vi "main.vi"() -> ()   [LabVIEW 2016]
doc: "Ezt a VI-t kell elindítani."
uses:
  adat.ctl
  <vilib>/Utility/file.llb/Write Delimited Spreadsheet (string).vi
panel:
  in  "1":enum32{""}(tab)
  in  "2":T1(tab)
  out "Waveform Graph":dbl[][](graph)
  out "XY Graph":cluster{dbl[], dbl[]}[](graph)
  out "Waveform Graph 2":dbl[][](graph)
  out "XY Graph 3":cluster{dbl[], dbl[]}[](graph)
  out "XY Graph 4":cluster{dbl[], dbl[]}[](graph)
  out "XY Graph 5":cluster{dbl[], dbl[]}[](graph)
  in  "Kiértékelés indítása":bool
  in  "Program leállítása":bool
  in  "Kilépés a programból":bool
  in  "Eredmények mentése":bool
  in  "Inicializálás":bool
  in  "Fájlbeolvasás":bool
  in  "Paraméterek betöltése":bool
  in  "Paraméterek mentése":bool
  in  "Kezelõpult":T2={"Filt_alsó"=750.0, "Filt_felsõ"=7400.0, "Optikai elem hossza (km)"=0.000445, "Referencia hullámhossz (nm)"=800.0, " Illesztendõ polinom fokszáma"=7, "Megjegyzések"="**********"}
  # "Az Ocean Optics spektográffal kapott 1D-s \nspektrális interferogramok FT alapú kiértékelése\n\nLabview-ban implementálta:\nTari Balázs"
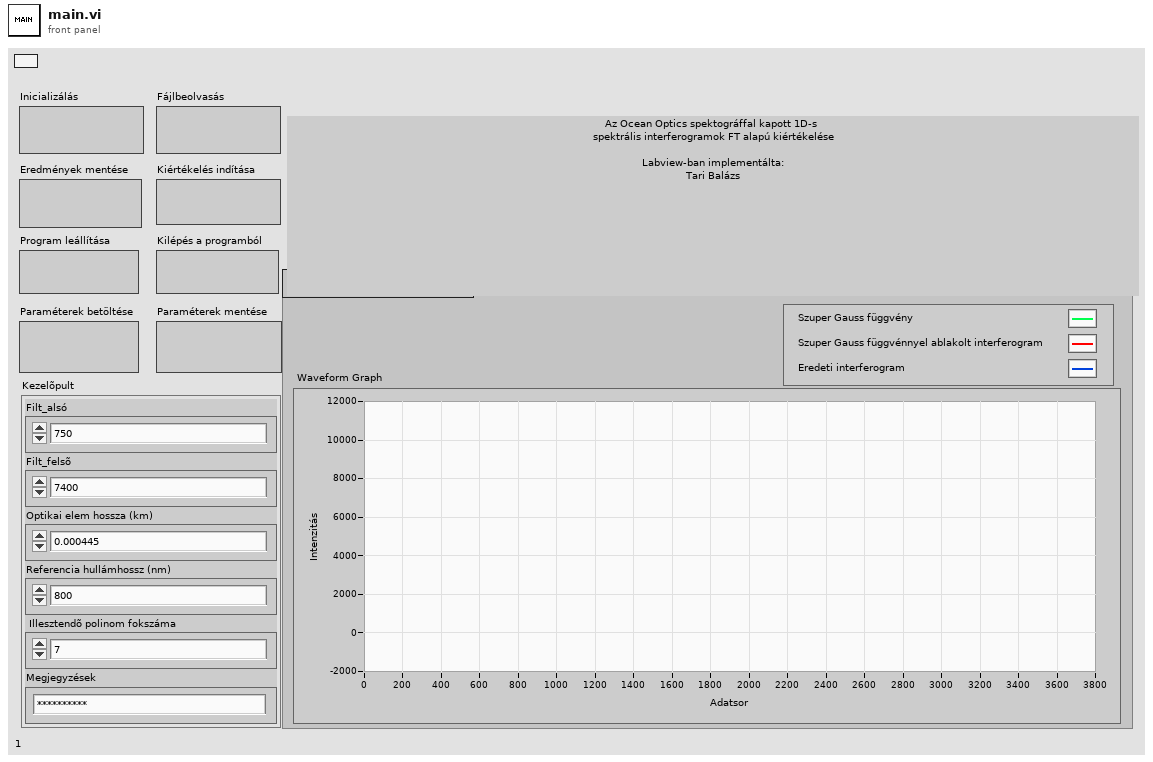
[diagram p1: front panel]
types:
  T1 = enum32{"Eredeti és módosított interferogram", "Megfordított interpolált és ablakolt interferogram", "Spektrum", "Fázis", "Fázisok összehasonlítása", "Diszperzió"}
  T2 = typedef "kezelõpult.ctl" = cluster{"Filt_alsó":dbl, "Filt_felsõ":dbl, "Optikai elem hossza (km)":dbl, "Referencia hullámhossz (nm)":dbl, " Illesztendõ polinom fokszáma":i32, "Megjegyzések":string}
  T3 = typedef "adat.ctl" = cluster{"Inicializálás":path, "Fájlbeolvasás":path, "Ix":dbl[], "dw":dbl, "Nw1":dbl, "Nw2":dbl, "FFT {X}":cdb[], "eredmények mentése":path}
  T4 = typedef "állapotok.ctl" = enum16{"init", "idle", "data load, filter, analysis", "filter", "analysis", "save", "save parameters", "load parameters", "stop"}
  T5 = enum16{"open", "replace", "create", "open or create", "replace or create", "replace or create with confirmation"}
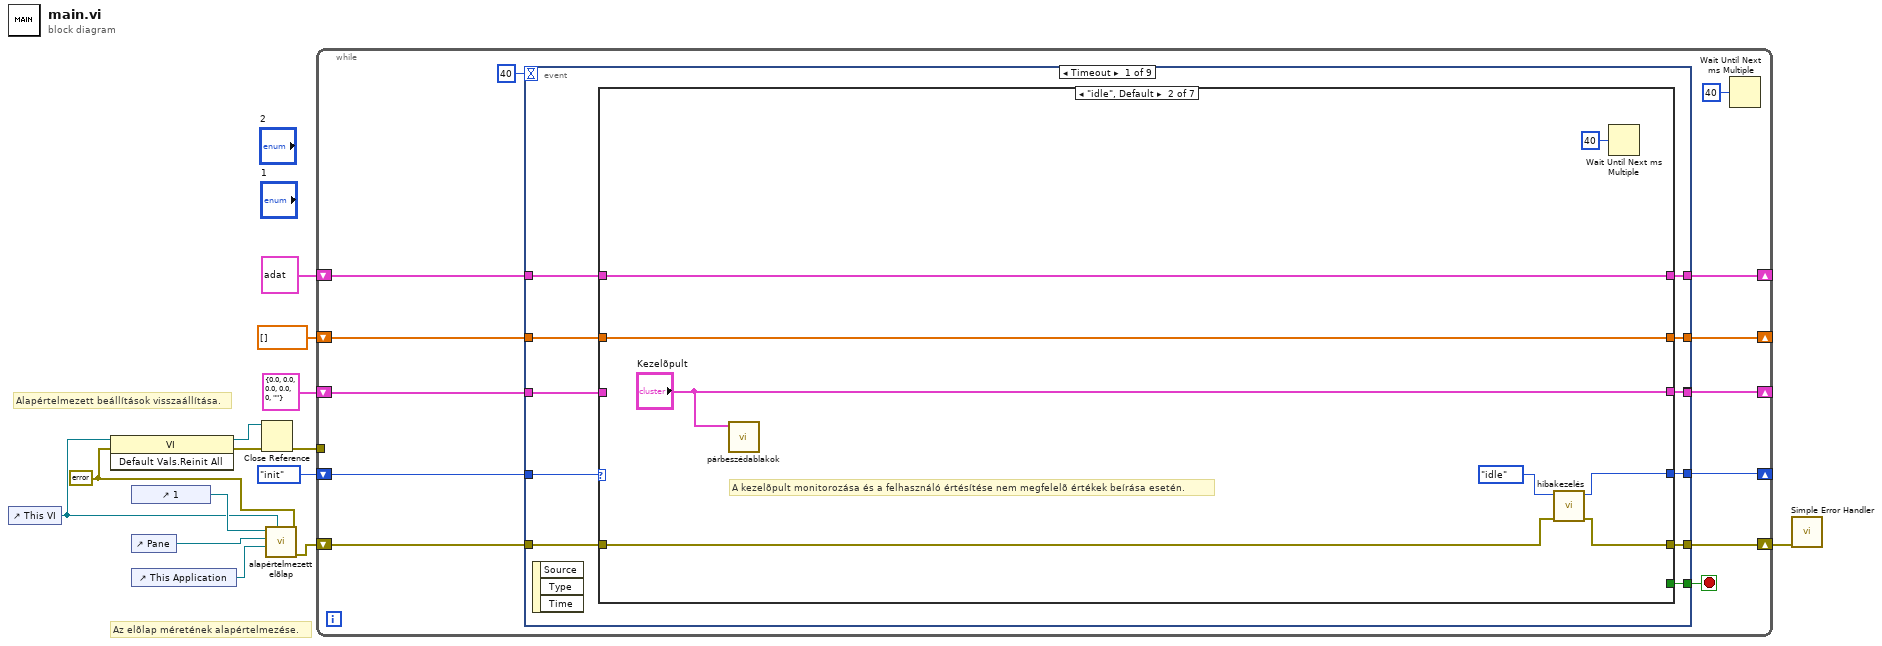
[diagram p0: block diagram]
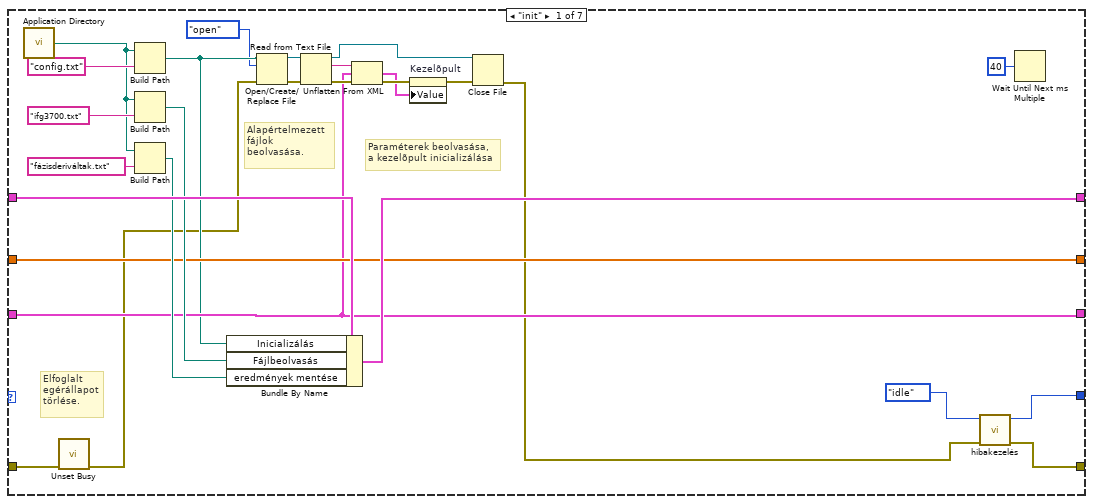
[diagram p2: hidden frame]
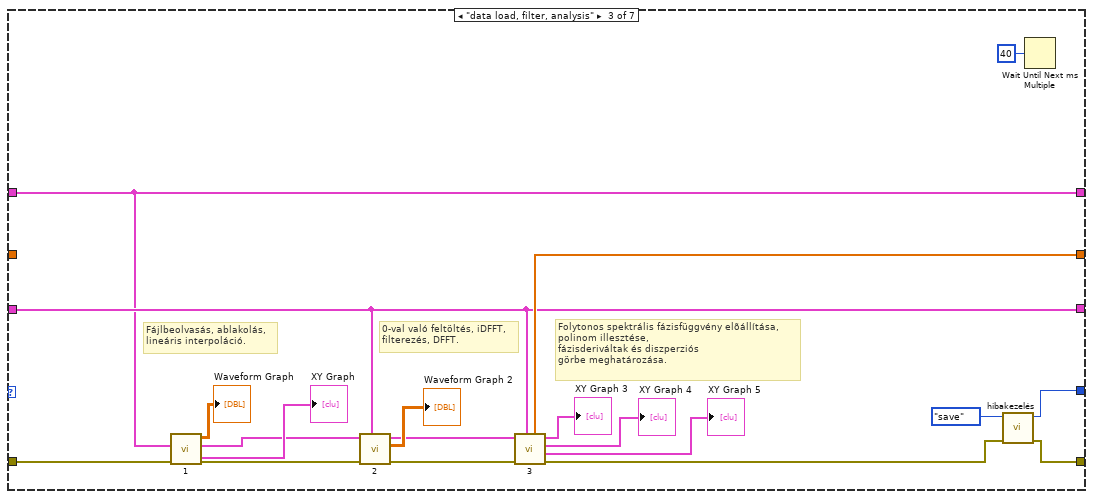
[diagram p3: hidden frame]
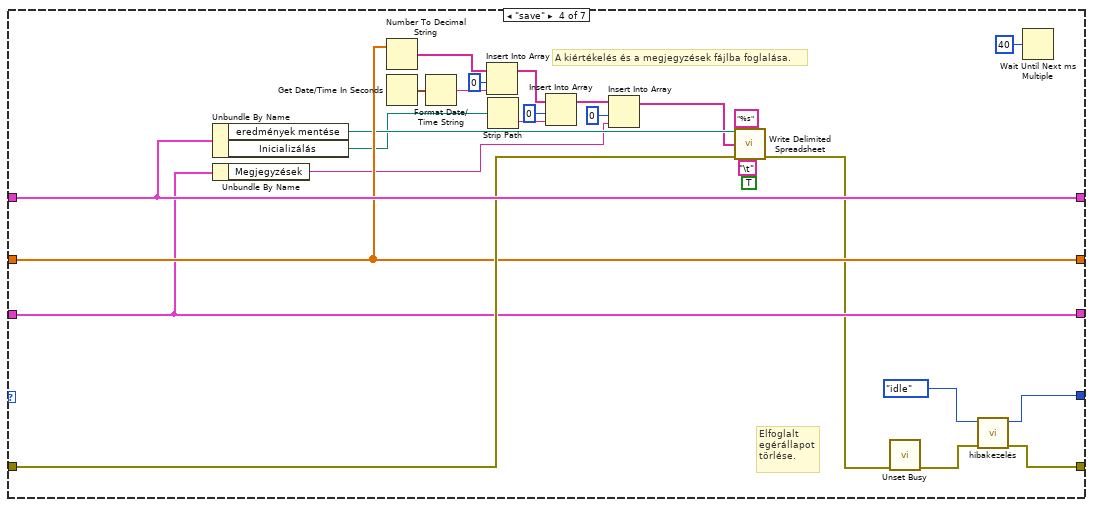
[diagram p4: hidden frame]
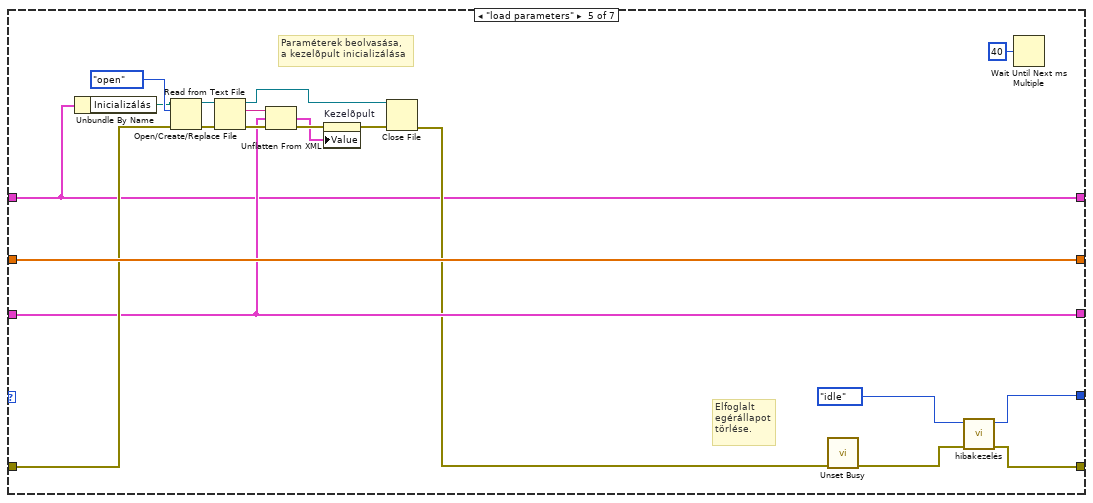
[diagram p5: hidden frame]
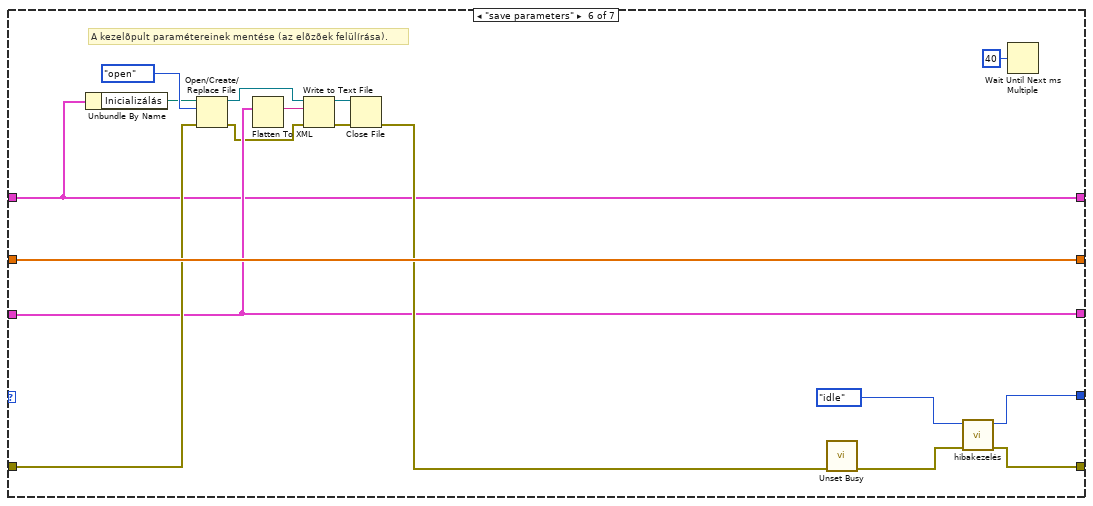
[diagram p6: hidden frame]
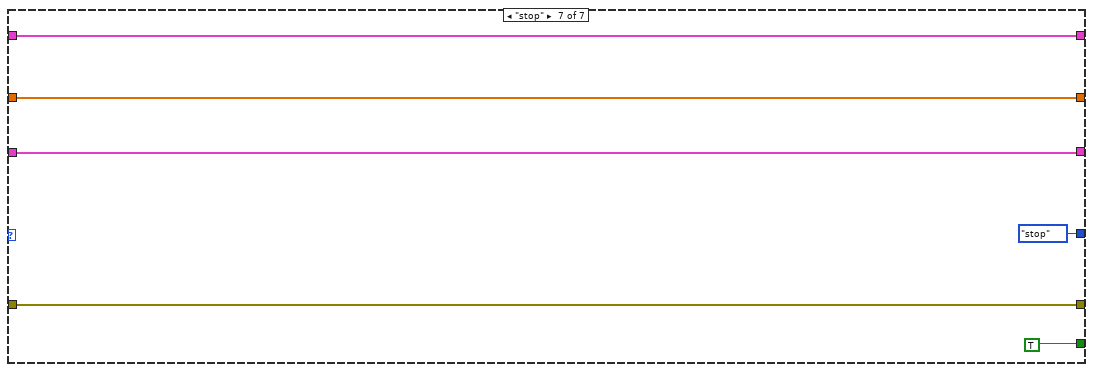
[diagram p7: hidden frame]
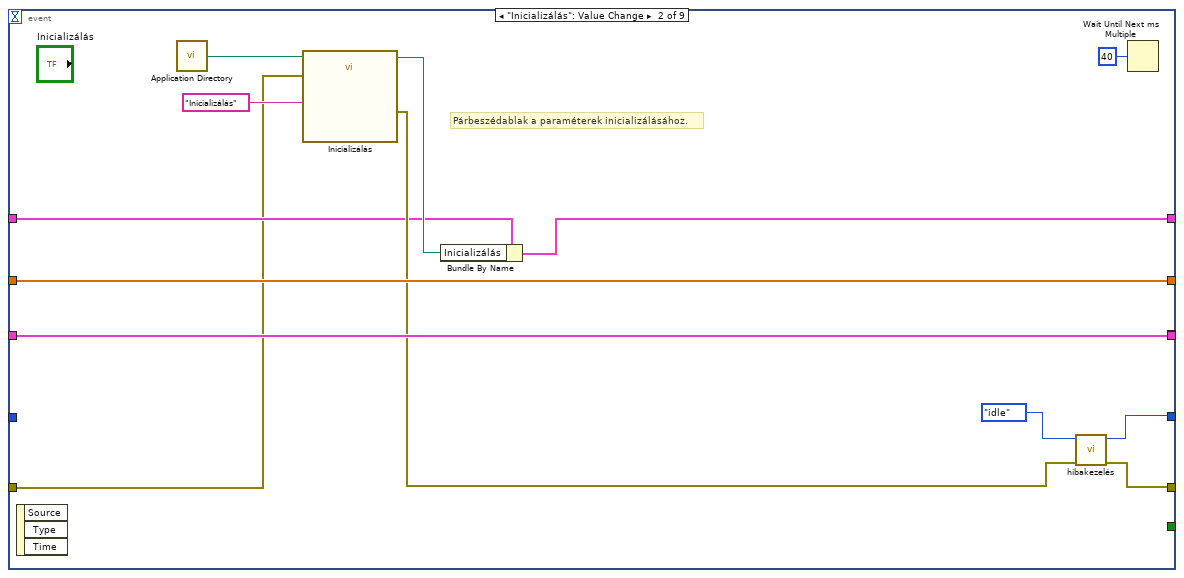
[diagram p8: hidden frame]
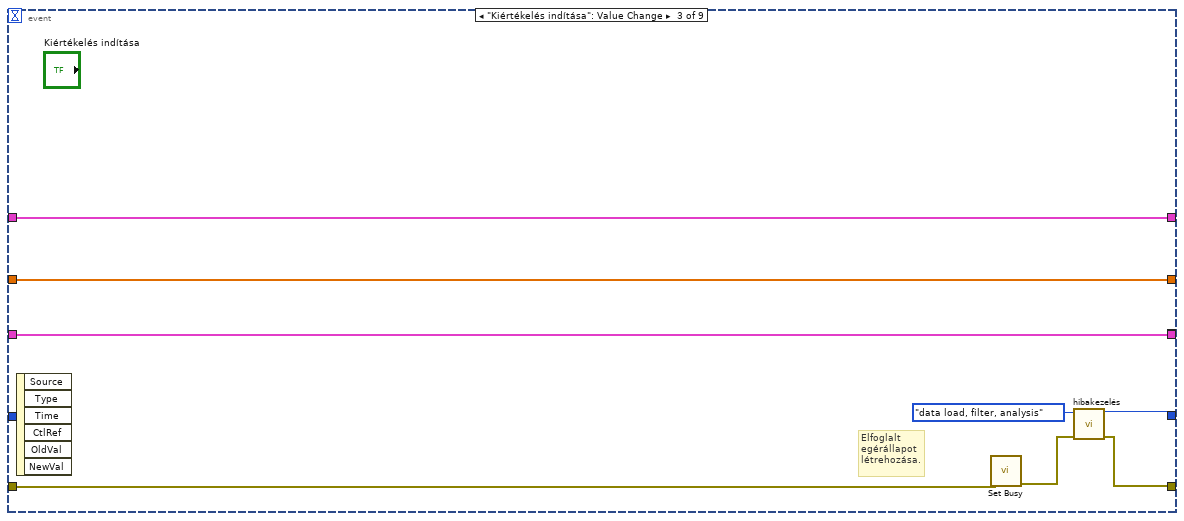
[diagram p9: hidden frame]
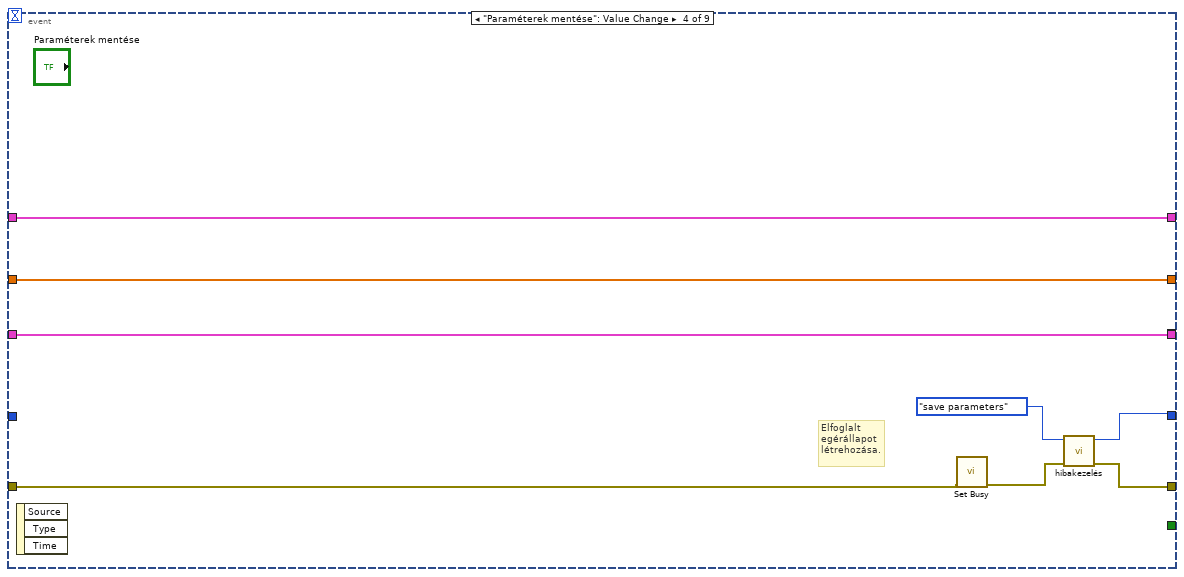
[diagram p10: hidden frame]
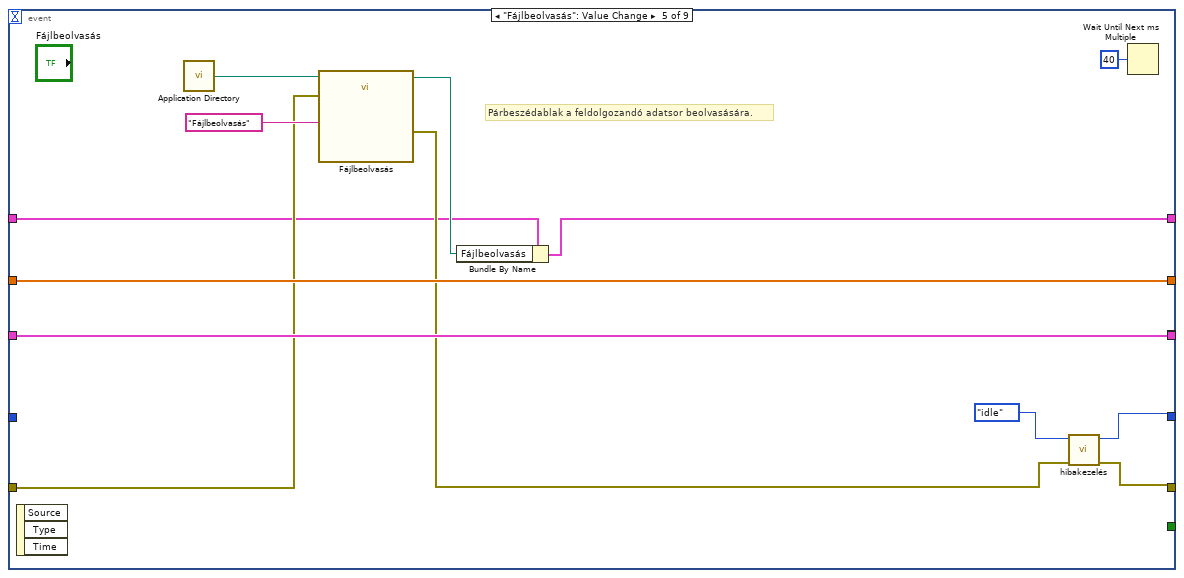
[diagram p11: hidden frame]
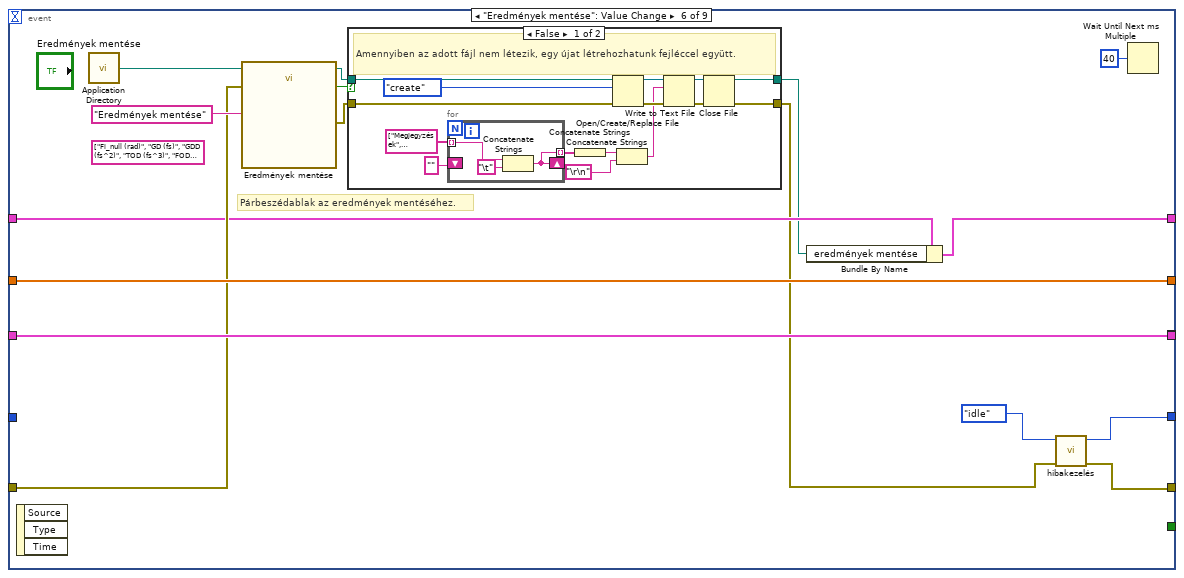
[diagram p12: hidden frame]
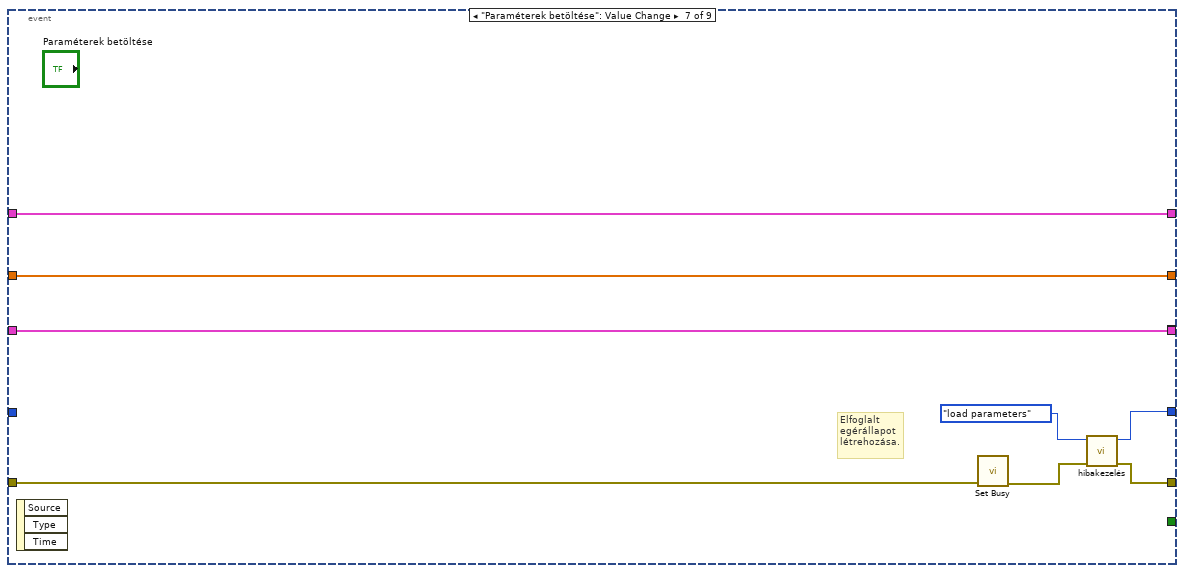
[diagram p14: hidden frame]
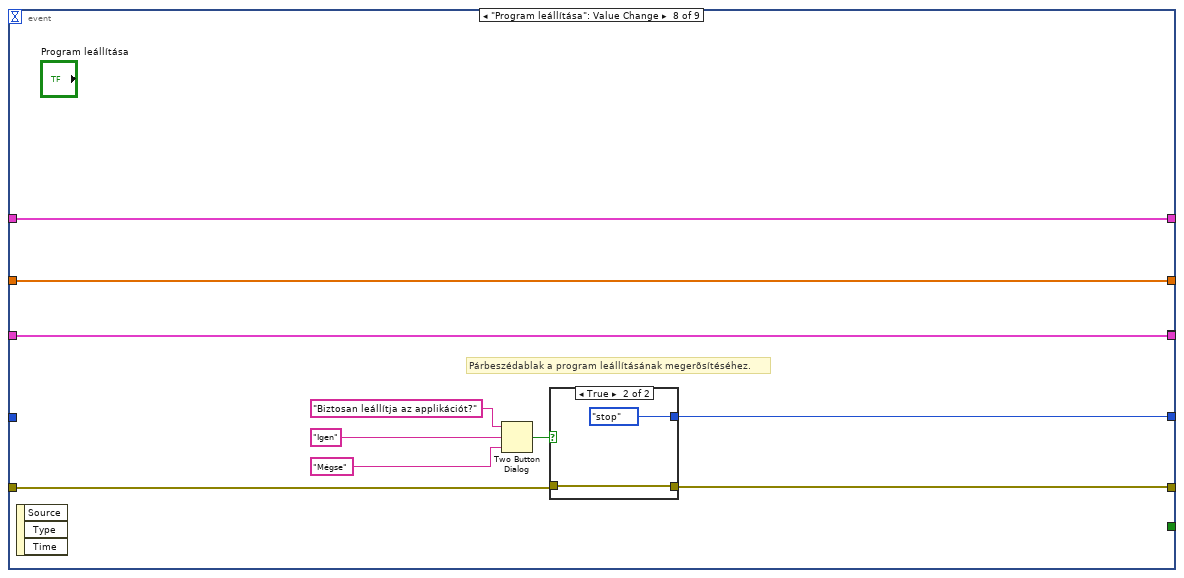
[diagram p15: hidden frame]
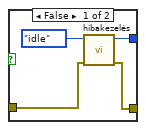
[diagram p16: hidden frame]
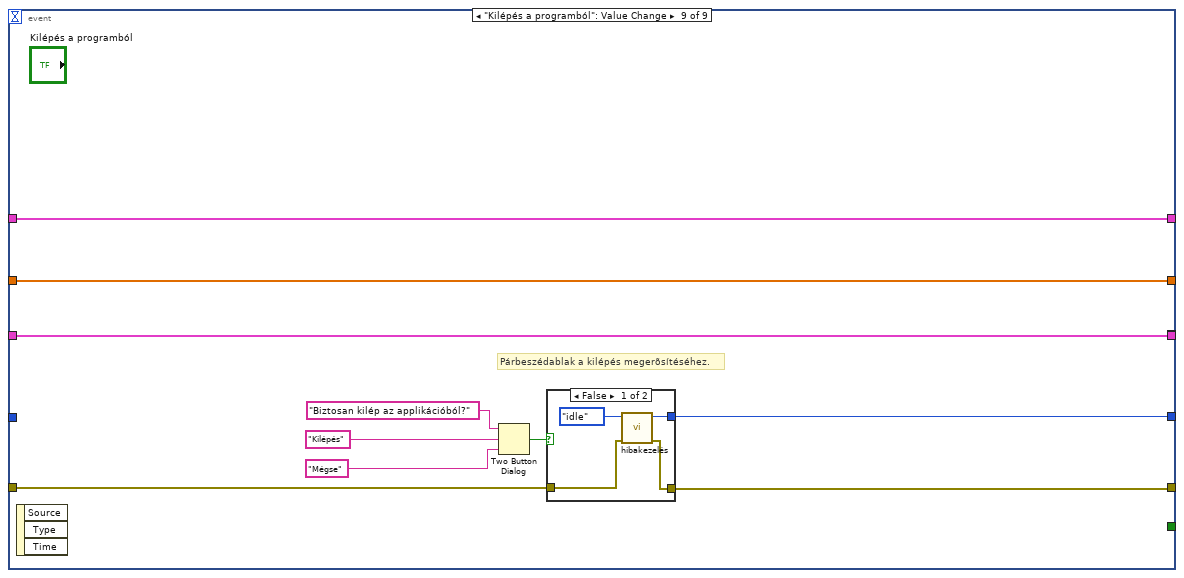
[diagram p17: hidden frame]
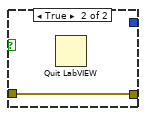
[diagram p18: hidden frame]
diagram:
  w6 = errorcluster {"status"=FALSE, "code"=0, "source"=""} ("error constant")
  # "Az elõlap méretének alapértelmezése."
  # "Alapértelmezett beállítások visszaállítása."
  n1 = control-ref of="This VI"() -> (w5:refnum<vi>)
  n2 = invoke class="VI" method="Default Vals.Reinit All"(reference=w5, error in=w6) -> (reference out=w3:refnum<vi>, error out=w4:errorcluster)  [unwired: 1 in, 1 out]
  n3 = control-ref of="1"() -> (w8:refnum<vi>)
  n4 = control-ref of="Pane"() -> (w7:refnum<vi>)
  n5 = control-ref of="This Application"() -> (w12:refnum<vi>)
  n6 = Close Reference(reference=w3, error in (no error)=w4) -> (error out=w1:errorcluster)
  n7 = call "alapértelmezett elõlap.vi"("error in (no error)"=w6, "VI Reference"=w5, "Application reference"=w12, "Pane Control"=w7, "TabControl in"=w8) -> ("error out"=w2:errorcluster)  [unwired: 6 in]
  n8 = while {
    shift-right: [w27] -> _
    shift-left: állapotok."init" -> [w17]
    shift-right: [w24] -> w11
    shift-left: w2 -> [w16]
    shift-right: [w23] -> _
    shift-left: T2 {"Filt_alsó"=0.0, "Filt_felsõ"=0.0, "Optikai elem hossza (km)"=0.0, "Referencia hullámhossz (nm)"=0.0, " Illesztendõ polinom fokszáma"=0, "Megjegyzések"=""} ("Kezelõpult") -> [w21]
    shift-right: [w20] -> _
    shift-left: T3 {"Inicializálás"=path "", "Fájlbeolvasás"=path "", "Ix"=[], "dw"=0.0, "Nw1"=0.0, "Nw2"=0.0, "FFT {X}"=[], "eredmények mentése"=path ""} ("adat") -> [w22]
    shift-right: [w19] -> _
    shift-left: dbl[] [] ("Fázisderiváltak") -> [w18]
    tunnel: w1 -> [_]
    stop <- w26 stop-if-true
    n9 = event shown="[0] Timeout" {
      selector: _ -> [_ _ _ _ _ _ _ _ _]
      dyn-events: _ -> [_ _ _ _ _ _ _ _ _]
      timeout: 40 -> [_ _ _ _ _ _ _ _ _]
      tunnel: w17 -> [w38 _ _ _ _ _ _ _ _]
      tunnel: [w37 w172 w180 w189 w201 w217 w246 w248 w264] -> w27
      tunnel: [w36 _ _ _ _ _ _ _ _] -> w26
      tunnel: [w34 w171 w179 w188 w200 w216 w245 w249 w267] -> w24
      tunnel: w16 -> [w35 w162 w177 w183 w195 w211 w240 w250 w268]
      tunnel: [w33 w169 w182 w185 w199 w215 _ w257 w265] -> w23
      tunnel: [w32 w165 w181 w187 w192 w205 w244 w256 w273] -> w20
      tunnel: w22 -> [w31 w164 w181 w187 w191 w210 w244 w256 w273]
      tunnel: w21 -> [w30 w169 w182 w185 w199 w215 w242 w257 w265]
      tunnel: [_ _ _ _ _ _ w242 _ _] -> _
      tunnel: [w29 w170 w178 w186 w198 w214 w243 w255 w266] -> w19
      tunnel: w18 -> [w28 w170 w178 w186 w198 w214 w243 w255 w266]
      event Timeout {
        n10 = event-data() -> ()  [unwired: 1 in, 3 out]
        n11 = case shown="\"idle\", Default" w38 {
          tunnel: [w65 w71 w89 w117 w136 w153 állapotok."stop" ("Enum out")] -> w37
          tunnel: [_ _ _ _ _ _ TRUE] -> w36
          tunnel: w35 -> [w40 w66 w88 w113 w122 w144 w161]
          tunnel: [w62 w70 w90 w116 w135 w152 w161] -> w34
          tunnel: [w48 "Kezelõpult" w80 w99 w121 w142 w157] -> w33
          tunnel: [w60 w67 w75 w115 w119 w141 w159] -> w32
          tunnel: w31 -> [w61 w67 w75 w115 w119 w141 w159]
          tunnel: w30 -> [w48 _ w80 w99 w121 w142 w157]
          tunnel: [w53 w68 w81 w112 w134 w145 w158] -> w29
          tunnel: w28 -> [w53 w68 _ w112 w134 w145 w158]
          frame "init" {
            # "Alapértelmezett \nfájlok\nbeolvasása."
            # "Paraméterek beolvasása,\na kezelõpult inicializálása"
            # "Elfoglalt\negérállapot\ntörlése."
            n12 = call <vilib>:"Application Directory.vi"() -> ("Application Directory"=w54:path)
            n13 = call <vilib>:"Unset Busy.vi"("error in (no error)"=w40) -> ("error out"=w39:errorcluster)  [unwired: 10 in]
            n14 = Build Path(base path=w54, name or relative path="config.txt") -> (appended path=w45:path)
            n15 = Build Path(base path=w54, name or relative path="ifg3700.txt") -> (appended path=w56:path)
            n16 = Build Path(base path=w54, name or relative path="fázisderiváltak.txt") -> (appended path=w55:path)
            n17 = Bundle By Name(cluster=w61, "Inicializálás"=w45, "Fájlbeolvasás"=w56, "eredmények mentése"=w55) -> (w60:T3)
            n18 = Open/Create/Replace File(file path (use dialog)=w45, error in=w39, operation (0:open)=T5."open") -> (refnum out=w46:refnum<file>, error out=w47:errorcluster)  [unwired: 3 in, 1 out]
            n19 = Read from Text File(file (use dialog)=w46, error in=w47) -> (refnum out=w42:refnum<file>, text=w49:string, error out=w52:errorcluster)  [unwired: 2 in, 1 out]
            n20 = Unflatten From XML(xml string=w49, type=w48, error in (no error)=w52) -> (value=w50:T2, error out=w51:errorcluster)
            n21 = property on="Kezelõpult" class="Clust (strict)"(error in=w51, "Value"=w50) -> (error out=w43:errorcluster)  [unwired: 1 in, 1 out]
            n22 = Close File(refnum=w42, error in=w43) -> (error out=w41:errorcluster)  [unwired: 1 out]
            n23 = call "hibakezelés.vi"("error in (no error)"=w41, "Enum in"=állapotok."idle") -> ("error out (no error)"=w62:errorcluster, "Enum out"=w65:T4)  [unwired: 8 in]
            n24 = Wait Until Next ms Multiple(millisecond multiple=u32 40 ("milliseconds to wait")) -> ()  [unwired: 1 out]
          }
          frame "idle", Default {
            # "A kezelõpult monitorozása és a felhasználó értésítése nem megfelelõ értékek beírása esetén."
            n25 = call "párbeszédablakok.vi"("kezelõpult"="Kezelõpult") -> ()  [unwired: 11 in]
            n26 = call "hibakezelés.vi"("error in (no error)"=w66, "Enum in"=állapotok."idle") -> ("error out (no error)"=w70:errorcluster, "Enum out"=w71:T4)  [unwired: 8 in]
            n27 = Wait Until Next ms Multiple(millisecond multiple=u32 40 ("milliseconds to wait")) -> ()  [unwired: 1 out]
          }
          frame "data load, filter, analysis" {
            # "Folytonos spektrális fázisfüggvény elõállítása, \npolinom illesztése, \nfázisderiváltak és diszperziós \ngörbe meghatározása."
            # "0-val való feltöltés, iDFFT,\nfilterezés, DFFT."
            # "Fájlbeolvasás, ablakolás, \nlineáris interpoláció."
            n28 = call "1.vi"("error in (no error)"=w88, "adat"=w75) -> ("error out"=w85:errorcluster, "adat"=w82:T3, "Waveform Graph"=→"Waveform Graph":dbl[][], "XY Graph"=→"XY Graph":cluster{dbl[], "yi":dbl[]}[])  [unwired: 6 in]
            n29 = call "2.vi"("Kezelõpult"=w80, "error in (no error)"=w85, "adat"=w82) -> ("error out"=w74:errorcluster, "Waveform Graph 2"=→"Waveform Graph 2":dbl[][], "adat"=w83:T3)  [unwired: 6 in]
            n30 = call "3.vi"("Kezelõpult"=w80, "error in (no error)"=w74, "adat"=w83) -> ("error out"=w79:errorcluster, "XY Graph 5"=→"XY Graph 5":cluster{dbl[], dbl[]}[], "XY Graph 4"=→"XY Graph 4":cluster{dbl[], dbl[]}[], "XY Graph 3"=→"XY Graph 3":cluster{dbl[], dbl[]}[], "Fázisderiváltak"=w81:dbl[])  [unwired: 4 in]
            n31 = call "hibakezelés.vi"("error in (no error)"=w79, "Enum in"=állapotok."save") -> ("error out (no error)"=w90:errorcluster, "Enum out"=w89:T4)  [unwired: 8 in]
            n32 = Wait Until Next ms Multiple(millisecond multiple=u32 40 ("milliseconds to wait")) -> ()  [unwired: 1 out]
          }
          frame "save" {
            # "A kiértékelés és a megjegyzések fájlba foglalása."
            # "Elfoglalt\negérállapot\ntörlése."
            n33 = Unbundle By Name(w115) -> ("eredmények mentése"=w101:path, "Inicializálás"=w100:path)
            n34 = Unbundle By Name(w99) -> ("Megjegyzések"=w96:string)
            n35 = Number To Decimal String(number=w112) -> (decimal integer string=w105:string[])  [unwired: 1 in]
            n36 = Get Date/Time In Seconds() -> (seconds since 1Jan1904=w106:timestamp)
            n37 = Format Date/Time String(seconds (now)=w106) -> (date/time string=w107:string)  [unwired: 2 in]
            n38 = Insert Into Array(array=w105, index=0, new element=w107) -> (w102:string[])
            n39 = Strip Path(path=w100) -> (name=w103:string)  [unwired: 1 out]
            n40 = Insert Into Array(array=w102, index=0, new element=w103) -> (w97:string[])
            n41 = Insert Into Array(array=w97, index=0, new element=w96) -> (w95:string[])
            n42 = call-poly <vilib>:"Write Delimited Spreadsheet.vi"("file path (dialog if empty)"=w101, "format (%s)"="%s", "1D data"=w95, "append to file? (new file:F)"=TRUE, "error in (no error)"=w113, "delimiter (\\t)"="\t") -> ("error out"=w93:errorcluster)  [unwired: 8 in, 1 out]
            n43 = call <vilib>:"Unset Busy.vi"("error in (no error)"=w93) -> ("error out"=w94:errorcluster)  [unwired: 10 in]
            n44 = call "hibakezelés.vi"("error in (no error)"=w94, "Enum in"=állapotok."idle") -> ("error out (no error)"=w116:errorcluster, "Enum out"=w117:T4)  [unwired: 8 in]
            n45 = Wait Until Next ms Multiple(millisecond multiple=u32 40 ("milliseconds to wait")) -> ()  [unwired: 1 out]
          }
          frame "load parameters" {
            # "Paraméterek beolvasása,\na kezelõpult inicializálása"
            # "Elfoglalt\negérállapot\ntörlése."
            n46 = Unbundle By Name(w119) -> ("Inicializálás"=w124:path)
            n47 = Open/Create/Replace File(file path (use dialog)=w124, error in=w122, operation (0:open)=T5."open") -> (refnum out=w128:refnum<file>, error out=w129:errorcluster)  [unwired: 3 in, 1 out]
            n48 = Read from Text File(file (use dialog)=w128, error in=w129) -> (refnum out=w125:refnum<file>, text=w130:string, error out=w133:errorcluster)  [unwired: 2 in, 1 out]
            n49 = Unflatten From XML(xml string=w130, type=w121, error in (no error)=w133) -> (value=w131:T2, error out=w132:errorcluster)
            n50 = property on="Kezelõpult" class="Clust (strict)"(error in=w132, "Value"=w131) -> (error out=w126:errorcluster)  [unwired: 1 in, 1 out]
            n51 = Close File(refnum=w125, error in=w126) -> (error out=w120:errorcluster)  [unwired: 1 out]
            n52 = call <vilib>:"Unset Busy.vi"("error in (no error)"=w120) -> ("error out"=w123:errorcluster)  [unwired: 10 in]
            n53 = call "hibakezelés.vi"("error in (no error)"=w123, "Enum in"=állapotok."idle") -> ("error out (no error)"=w135:errorcluster, "Enum out"=w136:T4)  [unwired: 8 in]
            n54 = Wait Until Next ms Multiple(millisecond multiple=u32 40 ("milliseconds to wait")) -> ()  [unwired: 1 out]
          }
          frame "save parameters" {
            # "A kezelõpult paramétereinek mentése (az elõzõek felülírása)."
            n55 = Unbundle By Name(w141) -> ("Inicializálás"=w146:path)
            n56 = Open/Create/Replace File(file path (use dialog)=w146, error in=w144, operation (0:open)=T5."open") -> (refnum out=w139:refnum<file>, error out=w140:errorcluster)  [unwired: 3 in, 1 out]
            n57 = Flatten To XML(anything=w142) -> (xml string=w150:string)
            n58 = Write to Text File(file (use dialog)=w139, text=w150, error in=w140) -> (refnum out=w148:refnum<file>, error out=w149:errorcluster)  [unwired: 1 in, 1 out]
            n59 = Close File(refnum=w148, error in=w149) -> (error out=w143:errorcluster)  [unwired: 1 out]
            n60 = call <vilib>:"Unset Busy.vi"("error in (no error)"=w143) -> ("error out"=w151:errorcluster)  [unwired: 10 in]
            n61 = call "hibakezelés.vi"("error in (no error)"=w151, "Enum in"=állapotok."idle") -> ("error out (no error)"=w152:errorcluster, "Enum out"=w153:T4)  [unwired: 8 in]
            n62 = Wait Until Next ms Multiple(millisecond multiple=u32 40 ("milliseconds to wait")) -> ()  [unwired: 1 out]
          }
          frame "stop" {
          }
        }
      }
      event "Inicializálás": Value Change {
        # "Párbeszédablak a paraméterek inicializálásához."
        n63 = event-data() -> ()  [unwired: 1 in, 3 out]
        n64 = call <vilib>:"Application Directory.vi"() -> ("Application Directory"=w168:path)
        n65 = call "Inicializálás"("start path"=w168, "button label"="Inicializálás", "error in"=w162) -> ("selected path"=w166:path, "error out"=w167:errorcluster)  [unwired: 9 in, 2 out]
        n66 = Bundle By Name(cluster=w164, "Inicializálás"=w166) -> (w165:T3)
        n67 = call "hibakezelés.vi"("error in (no error)"=w167, "Enum in"=állapotok."idle") -> ("error out (no error)"=w171:errorcluster, "Enum out"=w172:T4)  [unwired: 8 in]
        n68 = Wait Until Next ms Multiple(millisecond multiple=u32 40 ("milliseconds to wait")) -> ()  [unwired: 1 out]
      }
      event "Kiértékelés indítása": Value Change {
        # "Elfoglalt\negérállapot\nlétrehozása."
        n69 = event-data() -> ()  [unwired: 1 in, 6 out]
        n70 = call <vilib>:"Set Busy.vi"("error in (no error)"=w177) -> ("error out"=w176:errorcluster)  [unwired: 9 in, 1 out]
        n71 = call "hibakezelés.vi"("error in (no error)"=w176, "Enum in"=állapotok."data load, filter, analysis") -> ("error out (no error)"=w179:errorcluster, "Enum out"=w180:T4)  [unwired: 8 in]
      }
      event "Paraméterek mentése": Value Change {
        # "Elfoglalt\negérállapot\nlétrehozása."
        n72 = event-data() -> ()  [unwired: 1 in, 3 out]
        n73 = call <vilib>:"Set Busy.vi"("error in (no error)"=w183) -> ("error out"=w184:errorcluster)  [unwired: 9 in, 1 out]
        n74 = call "hibakezelés.vi"("error in (no error)"=w184, "Enum in"=állapotok."save parameters") -> ("error out (no error)"=w188:errorcluster, "Enum out"=w189:T4)  [unwired: 8 in]
      }
      event "Fájlbeolvasás": Value Change {
        # "Párbeszédablak a feldolgozandó adatsor beolvasására."
        n75 = event-data() -> ()  [unwired: 1 in, 3 out]
        n76 = call <vilib>:"Application Directory.vi"() -> ("Application Directory"=w197:path)
        n77 = call "Fájlbeolvasás"("start path"=w197, "button label"="Fájlbeolvasás", "error in"=w195) -> ("selected path"=w193:path, "error out"=w194:errorcluster)  [unwired: 9 in, 2 out]
        n78 = Bundle By Name(cluster=w191, "Fájlbeolvasás"=w193) -> (w192:T3)
        n79 = call "hibakezelés.vi"("error in (no error)"=w194, "Enum in"=állapotok."idle") -> ("error out (no error)"=w200:errorcluster, "Enum out"=w201:T4)  [unwired: 8 in]
        n80 = Wait Until Next ms Multiple(millisecond multiple=u32 40 ("milliseconds to wait")) -> ()  [unwired: 1 out]
      }
      event "Eredmények mentése": Value Change {
        (unwired) string[] ["Fi_null (rad)", "GD (fs)", "GDD (fs^2)", "TOD (fs^3)", "FOD (fs^4)", "QOD (fs^5)", "SOD (fs^6)", "SEOD (fs^7)", "EOD (fs^8)", "NOD (fs^9)", "TEOD (fs^10)"]
        # "Párbeszédablak az eredmények mentéséhez."
        n81 = event-data() -> ()  [unwired: 1 in, 3 out]
        n82 = call <vilib>:"Application Directory.vi"() -> ("Application Directory"=w212:path)
        n83 = call "Eredmények mentése"("start path"=w212, "button label"="Eredmények mentése", "error in"=w211) -> ("selected path"=w209:path, "exists"=w208:bool, "error out"=w207:errorcluster)  [unwired: 9 in, 1 out]
        n84 = case shown="False" w208 {
          tunnel: w209 -> [w233 w238]
          tunnel: w207 -> [w232 w239]
          tunnel: [w227 w239] -> w204
          tunnel: [w226 w238] -> w206
          frame False {
            # "Amennyiben az adott fájl nem létezik, egy újat létrehozhatunk fejléccel együtt."
            n85 = for {
              shift-right: [w235] -> _
              shift-left: "" -> [_]
              tunnel: string[] ["Megjegyzések", "Konfigurációs fájl", "A kiértékelés idõpontja ", "Fi_null (rad)", "GD (fs)", "GDD (fs^2)", "TOD (fs^3)", "FOD (fs^4)", "QOD (fs^5)", "SOD (fs^6)", "SEOD (fs^7)", "EOD (fs^8)", "NOD (fs^9)", "TEOD (fs^10)"] -> [w236] mode=indexing
              tunnel: [w235] -> w224 mode=indexing
              n86 = Concatenate Strings(w236, "\t") -> (w235:string)
            }
            n87 = Concatenate Strings(w224) -> (w223:string)
            n88 = Open/Create/Replace File(file path (use dialog)=w233, error in=w232, operation (0:open)=T5."create") -> (refnum out=w230:refnum<file>, error out=w231:errorcluster)  [unwired: 3 in, 1 out]
            n89 = Concatenate Strings(w223, "\r\n") -> (w221:string)
            n90 = Write to Text File(file (use dialog)=w230, text=w221, error in=w231) -> (refnum out=w228:refnum<file>, error out=w229:errorcluster)  [unwired: 1 in, 1 out]
            n91 = Close File(refnum=w228, error in=w229) -> (path=w226:path, error out=w227:errorcluster)
          }
          frame True {
            # "Amennyiben az adott fájl létezik, nem generálódik újabb fejléc függetlenül attól hogy van-e vagy nincs."
          }
        }
        n92 = Bundle By Name(cluster=w210, "eredmények mentése"=w206) -> (w205:T3)
        n93 = call "hibakezelés.vi"("error in (no error)"=w204, "Enum in"=állapotok."idle") -> ("error out (no error)"=w216:errorcluster, "Enum out"=w217:T4)  [unwired: 8 in]
        n94 = Wait Until Next ms Multiple(millisecond multiple=u32 40 ("milliseconds to wait")) -> ()  [unwired: 1 out]
      }
      event "Paraméterek betöltése": Value Change {
        # "Elfoglalt\negérállapot\nlétrehozása."
        n95 = event-data() -> ()  [unwired: 1 in, 3 out]
        n96 = call <vilib>:"Set Busy.vi"("error in (no error)"=w240) -> ("error out"=w241:errorcluster)  [unwired: 9 in, 1 out]
        n97 = call "hibakezelés.vi"("error in (no error)"=w241, "Enum in"=állapotok."load parameters") -> ("error out (no error)"=w245:errorcluster, "Enum out"=w246:T4)  [unwired: 8 in]
      }
      event "Program leállítása": Value Change {
        # "Párbeszédablak a program leállításának megerõsítéséhez."
        n98 = event-data() -> ()  [unwired: 1 in, 3 out]
        n99 = Two Button Dialog(message="Biztosan leállítja az applikációt?", 1:"Mégse" ("F button name (\"Cancel\")"), 2:"Igen" ("T button name (\"OK\")")) -> (T button?=w251:bool)
        n100 = case shown="True" w251 {
          tunnel: w250 -> [w260 w263]
          tunnel: [w259 w263] -> w249
          tunnel: [w258 állapotok."stop" ("Enum out")] -> w248
          frame False {
            n101 = call "hibakezelés.vi"("error in (no error)"=w260, "Enum in"=állapotok."idle") -> ("error out (no error)"=w259:errorcluster, "Enum out"=w258:T4)  [unwired: 8 in]
          }
          frame True {
          }
        }
      }
      event "Kilépés a programból": Value Change {
        # "Párbeszédablak a kilépés megerõsítéséhez."
        n102 = event-data() -> ()  [unwired: 1 in, 3 out]
        n103 = Two Button Dialog(message="Biztosan kilép az applikációból?", 1:"Mégse" ("F button name (\"Cancel\")"), 2:"Kilépés" ("T button name (\"OK\")")) -> (T button?=w269:bool)
        n104 = case shown="False" w269 {
          tunnel: w268 -> [w276 w278]
          tunnel: [w275 w278] -> w267
          tunnel: [w274 _] -> w264
          frame False {
            n105 = call "hibakezelés.vi"("error in (no error)"=w276, "Enum in"=állapotok."idle") -> ("error out (no error)"=w275:errorcluster, "Enum out"=w274:T4)  [unwired: 8 in]
          }
          frame True {
            n106 = Quit LabVIEW() -> ()  [unwired: 1 in]
          }
        }
      }
    }
    n107 = Wait Until Next ms Multiple(millisecond multiple=u32 40 ("milliseconds to wait")) -> ()  [unwired: 1 out]
  }
  n108 = call <vilib>:"Simple Error Handler.vi"("error in (no error)"=w11) -> ()  [unwired: 4 in, 5 out]
